vi "Configure Trigger (Video).vi"(0 "VISA resource name":refnum<visa-resource-name>, 1 "Line (1)":dbl=1.0, 2 "Trigger Level (0)":dbl, 5 "Source (1: Channel 1)":i32(ring)=1 items=["Channel 1"=1, "Channel 2"=2, "Channel 3"=3, "Channel 4"=4], 7 "Polarity (0: Positive)":i32(ring) items=["Positive", "Negative"], 9 "Mode (2: Any Field)":i32(ring)=2 items=["AnyLine", "GotoLine", "AnyFiled", "EvenFiled", "OddFiled"], 11 "error in (no error)":errorcluster, 12 "Video Standard (0: NTSC)":i32(ring) items=["NTSC", "Palsecam", "Secam"]) -> (4 "VISA resource name out":refnum<visa-resource-name>, 15 "error out":errorcluster)   [LabVIEW 2015, in "ZhiYuan ZDS Series for TCP.lvlib"]
doc: "This VI configures the setting for video trigger."
uses:
  ZhiYuan ZDS Series for TCP.lvlib
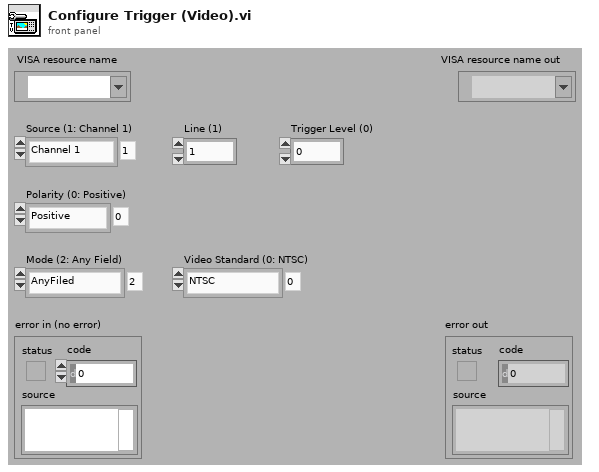
[diagram p1: front panel]
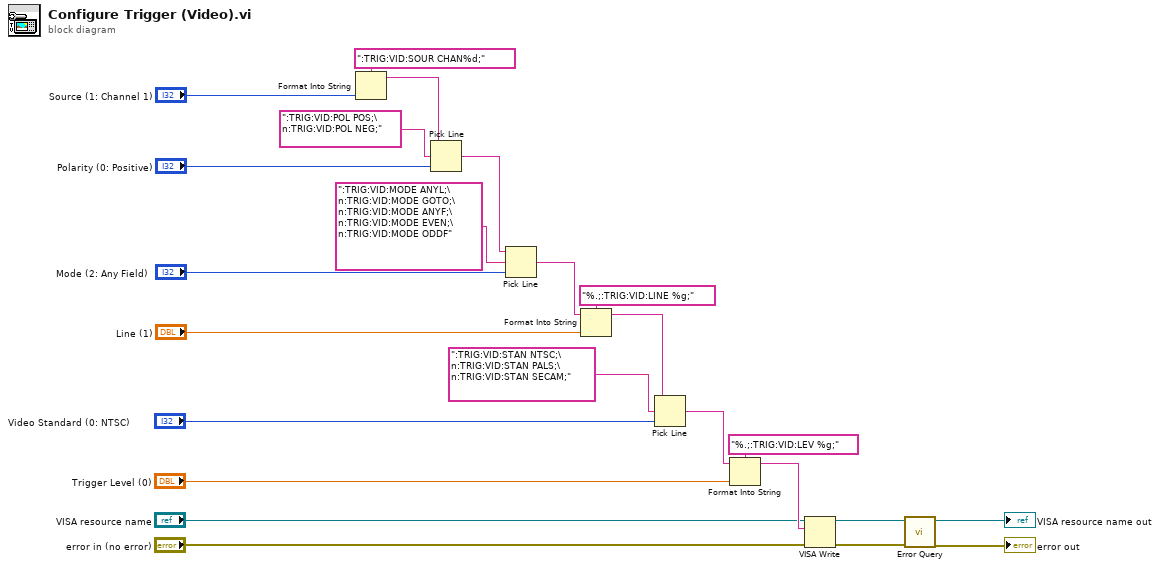
[diagram p0: block diagram]
diagram:
  n1 = Format Into String(format string=":TRIG:VID:SOUR CHAN%d;", "Source (1: Channel 1)") -> (resulting string=w20:string)  [unwired: 2 in, 1 out]
  n2 = Pick Line(string ("")=w20, multi-line string=":TRIG:VID:POL POS;\n:TRIG:VID:POL NEG;", line index="Polarity (0: Positive)") -> (output string=w17:string)
  n3 = Pick Line(string ("")=w17, multi-line string=":TRIG:VID:MODE ANYL;\n:TRIG:VID:MODE GOTO;\n:TRIG:VID:MODE ANYF;\n:TRIG:VID:MODE EVEN;\n:TRIG:VID:MODE ODDF", line index="Mode (2: Any Field)") -> (output string=w16:string)
  n4 = Format Into String(format string="%.;:TRIG:VID:LINE %g;", initial string=w16, "Line (1)") -> (resulting string=w11:string)  [unwired: 1 in, 1 out]
  n5 = Pick Line(string ("")=w11, multi-line string=":TRIG:VID:STAN NTSC;\n:TRIG:VID:STAN PALS;\n:TRIG:VID:STAN SECAM;", line index="Video Standard (0: NTSC)") -> (output string=w10:string)
  n6 = Format Into String(format string="%.;:TRIG:VID:LEV %g;", initial string=w10, "Trigger Level (0)") -> (resulting string=w7:string)  [unwired: 1 in, 1 out]
  n7 = VISA Write(VISA resource name="VISA resource name", write buffer=w7, error in (no error)="error in (no error)") -> (VISA resource name out=w4:refnum<visa-resource-name>, error out=w3:errorcluster)  [unwired: 1 out]
  n8 = call "Error Query.vi"("error in (no error)"=w3, "VISA resource name"=w4) -> ("error out"=→"error out":errorcluster, "VISA resource name out"=→"VISA resource name out":refnum<visa-resource-name>)  [unwired: 6 in, 2 out]
